vi "SE Initialization VI.vi"(8 "error in (no error)":errorcluster, 10 "Custom XML":string, 11 "Device Item Ref in":T1 format="%.0x") -> (0 "error out":errorcluster, 3 "Device Item Ref out":T1 format="%.0x")   [LabVIEW 2017, in "PXImc System Explorer.lvlib"]
uses:
  PXImc System Explorer.lvlib
  <vilib>/NI Veristand/Custom Device API/Custom Device Item Ref.ctl
  <vilib>/NI Veristand/Custom Device API/Custom Device Channel Type.ctl
  Shared/Channel.ctl
  Shared/Constants.vi
  Shared/PXImc Shared.lvlib
  <vilib>/NI VeriStand/Custom Device API/Custom Device API.lvlib
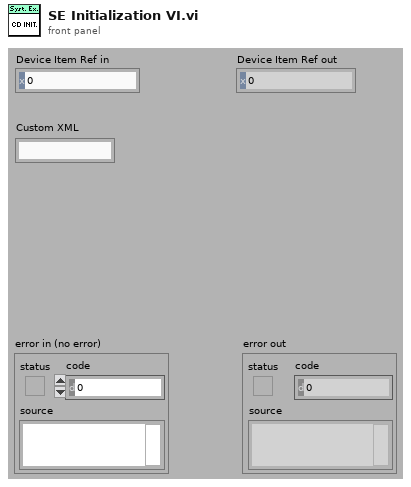
[diagram p1: front panel]
types:
  T1 = typedef "Custom Device API.lvlib/Custom Device Item Ref.ctl" = u64
  T2 = typedef "Custom Device API.lvlib/Custom Device Channel Type.ctl" = enum16{"Input", "Output"}
  T3 = typedef "PXImc Shared.lvlib/Channel.ctl" = cluster{"Name":string, "Units":string, "Default":dbl, "Description":string}
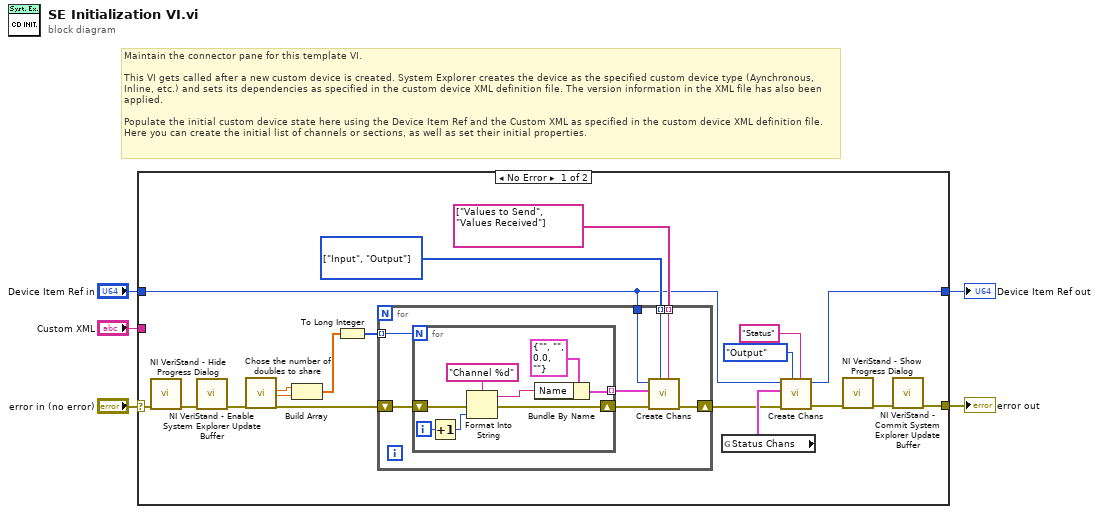
[diagram p0: block diagram]
diagram:
  # "Maintain the connector pane for this template VI.\n\nThis VI gets called after a new custom device is created. System Explorer creates the device as the specified custom device type (Aynchronous, Inline, etc.) and sets its dependencies as specified in the custom device XML definition file. The version information in the XML file has also been applied.\n\nPopulate the initial custom device state here using the Device Item Ref and the Custom XML as specified in the custom device XML definition file. Here you can create the initial list of channels or sections, as well as set their initial properties."
  n1 = case shown="No Error" "error in (no error)" {
    selector: "error in (no error)" -> [w17 w42]
    tunnel: [w12 w42] -> w5
    tunnel: [w24 w41] -> w3
    tunnel: "Device Item Ref in" -> [w6 w41]
    tunnel: "Custom XML" -> [_ _]
    frame No Error {
      w9 = T2[] [enum."Input", enum."Output"] items=["Input", "Output"]
      n2 = call <vilib>:"NI VeriStand - Hide Progress Dialog.vi"("error in (no error)"=w17) -> ("error out"=w16:errorcluster)  [unwired: 10 in]
      n3 = call <vilib>:"NI VeriStand - Enable System Explorer Update Buffer.vi"("error in (no error)"=w16) -> ("error out"=w15:errorcluster)  [unwired: 10 in]
      n4 = call "Chose the number of doubles to share"("error in (no error)"=w15) -> ("Doubles to receive"=w20:dbl, "Doubles to send"=w21:dbl, "error out"=w18:errorcluster)  [unwired: 15 in, 1 out]
      n5 = Build Array(w20, w21) -> (w19:dbl[])
      n6 = To Long Integer(number=w19) -> (32bit integer=w7:i32[])
      n7 = for {
        tunnel: w7 -> [w25] mode=indexing
        shift-right: [w31] -> w11
        shift-left: w18 -> [w32]
        tunnel: string[] ["Values to Send", "Values Received"] -> [w28] mode=indexing
        tunnel: w9 -> [w27] mode=indexing
        tunnel: w6 -> [w26]
        n8 = for {
          N: w25 -> [_]
          shift-right: [w36] -> w30
          shift-left: w32 -> [w34]
          tunnel: [w39] -> w29 mode=indexing
          i -> [w38]
          n9 = Increment(x=w38) -> (x+1=w33:i32)
          n10 = Format Into String(format string="Channel %d" ("string"), error in=w34, w33) -> (resulting string=w35:string, error out=w36:errorcluster)  [unwired: 1 in]
          n11 = Bundle By Name(cluster=T3 {"Name"="", "Units"="", "Default"=0.0, "Description"=""} ("Channel"), "Name"=w35) -> (w39:T3)
        }
        n12 = call "Create Chans.vi"("New Section Name (none)"=w28, "Type"=w27, "error in (no error)"=w30, "Channels"=w29, "Section Ptr"=w26) -> ("error out"=w31:errorcluster)  [unwired: 5 in, 1 out]
      }
      n13 = global read "Constants.vi" "Status Chans"() -> (w23:T3[])
      n14 = call "Create Chans.vi"("New Section Name (none)"="Status", "Type"=Custom_Device_Channel_Type."Output", "error in (no error)"=w11, "Channels"=w23, "Section Ptr"=w6) -> ("error out"=w14:errorcluster, "Section Ptr dup"=w24:T1)  [unwired: 5 in]
      n15 = call <vilib>:"NI VeriStand - Show Progress Dialog.vi"("error in (no error)"=w14) -> ("error out"=w13:errorcluster)  [unwired: 10 in]
      n16 = call <vilib>:"NI VeriStand - Commit System Explorer Update Buffer.vi"("error in (no error)"=w13) -> ("error out"=w12:errorcluster)  [unwired: 10 in]
    }
    frame Error {
    }
  }
  "error out" <- w5
  "Device Item Ref out" <- w3
